vi "Get valid data from parameters table.vi"(11 "Parameter Full Row Data":string[](array[string])) -> (3 "array w/ subset deleted":string[](array[string]))   [LabVIEW 2015, in "SQLite.lvclass"]
uses:
  SQLite.lvclass
panel:
  out "array w/ subset deleted 2":string[](array[string])
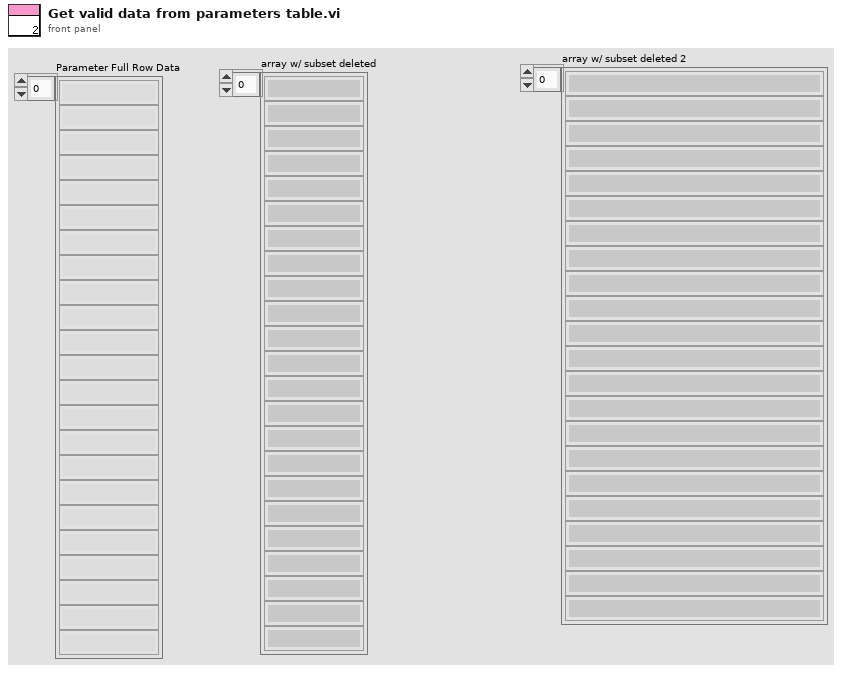
[diagram p1: front panel]
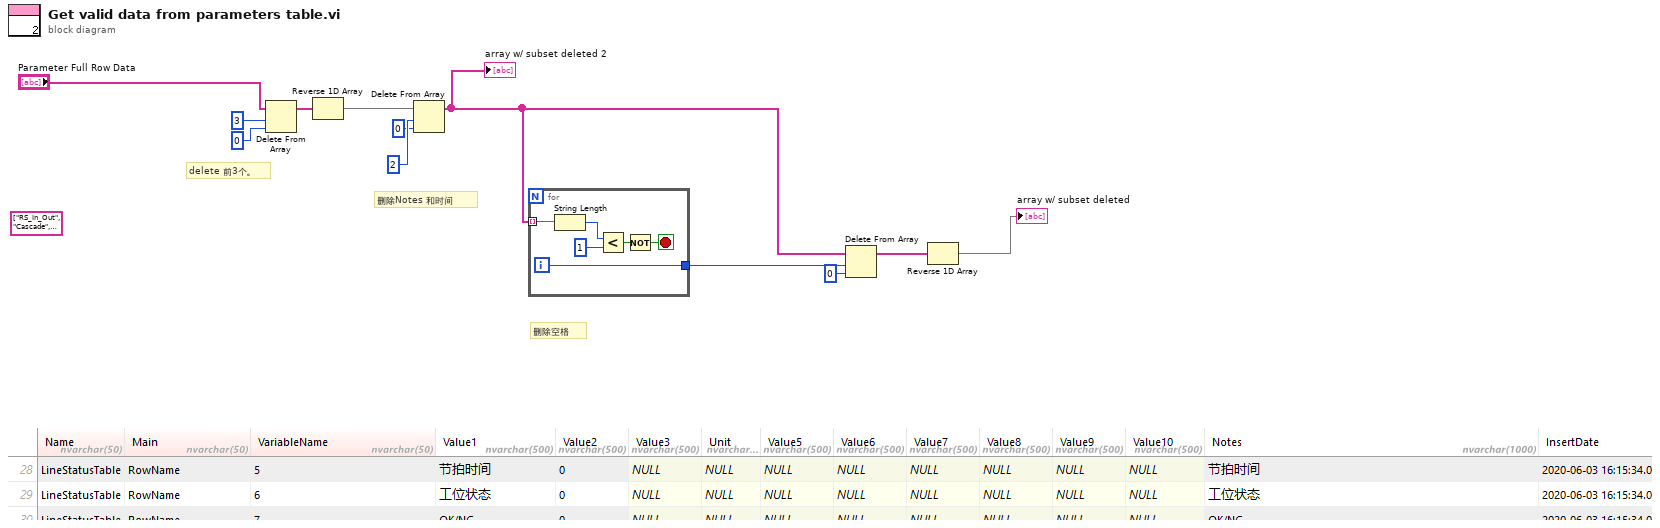
[diagram p0: block diagram]
diagram:
  (unwired) string[] ["RS_In_Out", "Cascade", "0", "OP070-1", "OP060F", "OP045F", "OP040F", "", "", "", "", "", "", "线外工位具有层级的依赖关系，工位1的条码与工位2绑定，工位2与工位3绑定，工位3与线内工位绑定。需要依次解析更新对应线外工位的MainBarcode", "2020-06-03 16:15:34"] ("Parameter Full Row Data")
  # "删除空格"
  # "删除Notes 和时间"
  # "delete 前3个。"
  n1 = Delete From Array(array="Parameter Full Row Data", length=3, index=0) -> (array with subset deleted=w10:string[])  [unwired: 1 out]
  n2 = Reverse 1D Array(array=w10) -> (reversed array=w4:string[])
  n3 = Delete From Array(array=w4, length=2, index=0) -> (array with subset deleted=w1:string[])  [unwired: 1 out]
  "array w/ subset deleted 2" <- w1
  n4 = for {
    tunnel: w1 -> [w18] mode=indexing
    tunnel: [w13] -> w9
    i -> [w13]
    stop <- w14 stop-if-true
    n5 = String Length(string=w18) -> (length=w17:i32)
    n6 = Less?(x=w17, y=1) -> (x < y?=w15:bool)
    n7 = Not(x=w15) -> (.not. x?=w14:bool)
  }
  n8 = Delete From Array(array=w1, length=w9, index=0) -> (array with subset deleted=w7:string[])  [unwired: 1 out]
  n9 = Reverse 1D Array(array=w7) -> (reversed array=→"array w/ subset deleted":string[])
